vi "Tool Data.TestLauncher.vi"() -> ()   [LabVIEW 2019, in "Tool Data.lvclass"]
uses:
  Tool Data.lvclass
  <vilib>/JKI/JKI SMO/SMO/Typedefs/SMOState --Enum.ctl
  C:/Program Files (x86)/National Instruments/LabVIEW 2019/vi.lib/JKI/JKI SMO/SMO/SMO.lvclass
  Typedefs/PrivateEvents--Tool Data.Update Objects.ctl
  Settings/Setting Database/Typedefs/PublicEvents--Setting Database.PathsUpdated.ctl
  Settings/Path Settings/Path Settings.lvclass
  Settings/Setting Database/Typedefs/PublicEvents--Setting Database.RectanglesUpdated.ctl
  Settings/Rectangle Settings/Rectangle Settings.lvclass
  Settings/Setting Database/Typedefs/PublicEvents--Setting Database.FunnelsUpdated.ctl
  Settings/Funnel Settings/Funnel Settings.lvclass
  Settings/Setting Database/Typedefs/PublicEvents--Setting Database.DotsUpdated.ctl
  Settings/Dot Settings/Dot Settings.lvclass
  Parse/ParsePaths/Path.lvclass
  Parse/Rectangle/Rectangle.lvclass
  Parse/Image/SVGImage.lvclass
  Parse/Dot/Dot.lvclass
  <vilib>/JKI/JKI SMO/SMO/SMO.lvclass/SMO.ctl
  Tool Data.lvclass/Tool Data.ctl
  <vilib>/JKI/JKI SMO/SMO/Private/ReftoDVR--SMO.vi
  <vilib>/JKI/JKI SMO/SMO/SMO.lvclass
  Settings/Setting Database/Setting Database.lvclass
  Parse/PathCommands.Moveto/PathCommands.MoveTo.lvclass
  Parse/PathCommands.LineTo/PathCommands.LineTo.lvclass
  Parse/PathCommands.CurveTo/PathCommands.CurveTo.lvclass
  Parse/PathCommands.ClosePath/PathCommands.ClosePath.lvclass
  Parse/CSSProperties/CSSProperties.lvclass
  Parse/Transform.Translate/Transform.Translate.lvclass
  Parse/Transform.Matrix/Transform.Matrix.lvclass
panel:
  out "XY Graph":cluster{"X":dbl, "Y":dbl}[](graph)
  out "Paths":i32
  out "Rects":i32
  out "Funnels":i32
  out "Dots":i32
  in  "Send":bool
  out "SMO State":T1
  out "error out":errorcluster
  in  "Stop":bool
  # "Basic SMO Test Launcher"
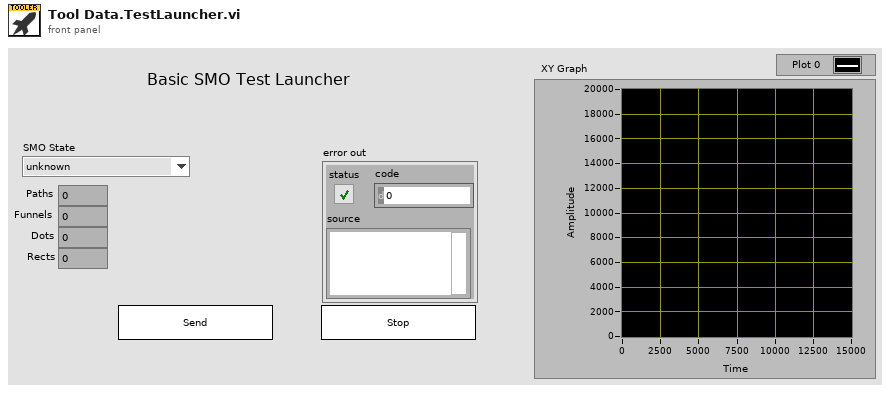
[diagram p1: front panel]
types:
  T1 = typedef "SMO.lvclass/SMOState --Enum.ctl" = enum16{"unknown", "Created", "Started", "Stopped"}
  T2 = typedef "Tool Data.lvclass/PrivateEvents--Tool Data.Update Objects.ctl" = cluster{"Settings":cluster{"Paths":T3, "Rectangles":T4, "Funnels":T5, "Dots":T6}, "Data":cluster{"Paths":refnum<class "Path.lvclass">[], "Rectangles":refnum<class "Rectangle.lvclass">[], "SVGImage":refnum<class "SVGImage.lvclass">, "Dots":refnum<class "Dot.lvclass">[], "Funnels":refnum<class "Path.lvclass">[]}}
  T3 = typedef "Setting Database.lvclass/PublicEvents--Setting Database.PathsUpdated.ctl" = refnum<class "Path Settings.lvclass">[]
  T4 = typedef "Setting Database.lvclass/PublicEvents--Setting Database.RectanglesUpdated.ctl" = refnum<class "Rectangle Settings.lvclass">[]
  T5 = typedef "Setting Database.lvclass/PublicEvents--Setting Database.FunnelsUpdated.ctl" = refnum<class "Funnel Settings.lvclass">[]
  T6 = typedef "Setting Database.lvclass/PublicEvents--Setting Database.DotsUpdated.ctl" = refnum<class "Dot Settings.lvclass">[]
  T7 = cluster{"Paths":T3, "Rectangles":T4, "Funnels":T5, "Dots":T6}
  T8 = cluster{"Paths":refnum<class "Path.lvclass">[], "Rectangles":refnum<class "Rectangle.lvclass">[], "SVGImage":refnum<class "SVGImage.lvclass">, "Dots":refnum<class "Dot.lvclass">[]}
  T9 = typedef "SMO.lvclass/Public Events.ctl" = cluster{"Error":refnum<user-event>, "State":refnum<user-event>, "Reserve State":refnum<user-event>}
  T10 = typedef "Tool Data.lvclass/PublicEvents--Cluster.ctl" = cluster{"Objects Updated":refnum<user-event>}
  T11 = cluster{"Event Registration Refnum":refnum<event-registration>}
  T12 = typedef "Relay-Box.lvclass/Resistor--enum.ctl" = enum16{"open", "discharge tip", "0 ohms", "100k ohm", "10M ohm", "1G ohm"}
  T13 = cluster{"Name":string, "Litho":cluster{"X":dbl, "Y":dbl, "Speed":dbl, "Voltage":dbl}[], "Set Resistance":T12, "Meta":variant}[]
  T14 = cluster{"X":dbl, "Y":dbl, "Speed":dbl, "Voltage":dbl}[]
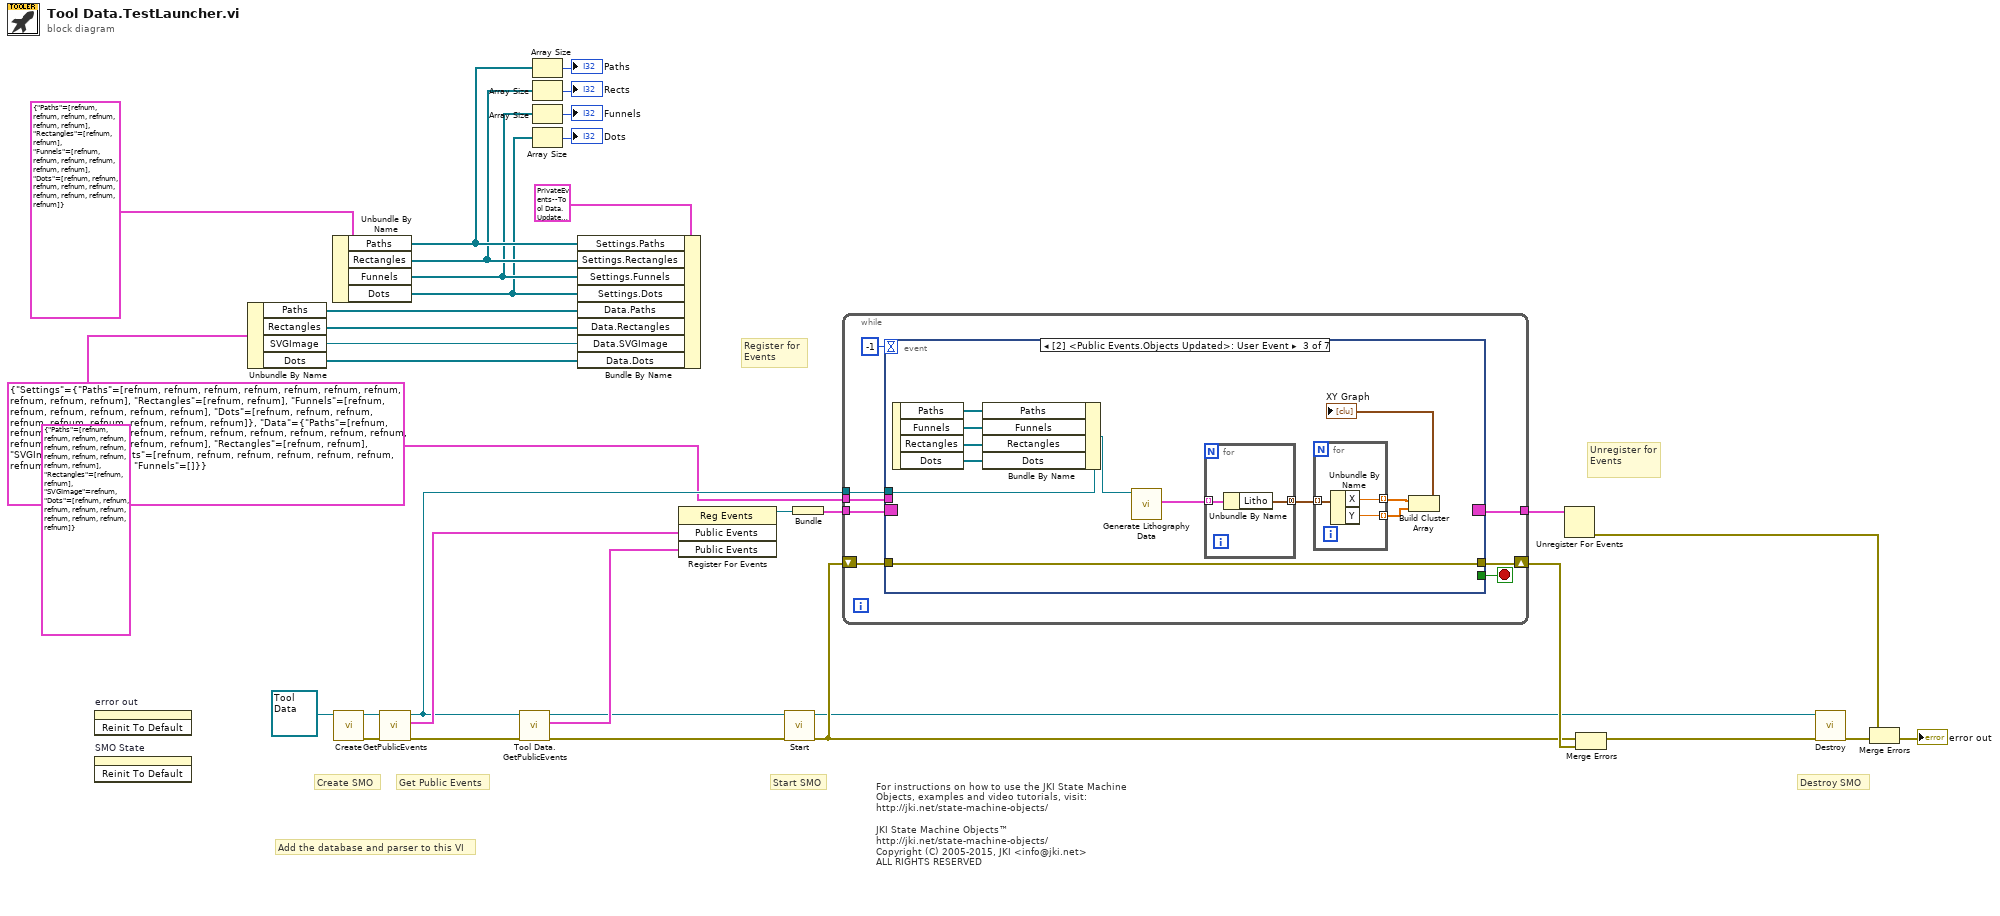
[diagram p0: block diagram]
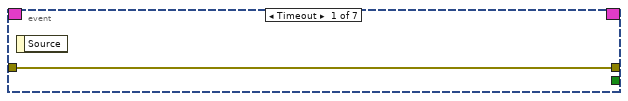
[diagram p2: hidden frame]
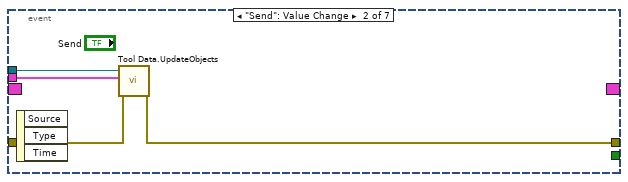
[diagram p3: hidden frame]
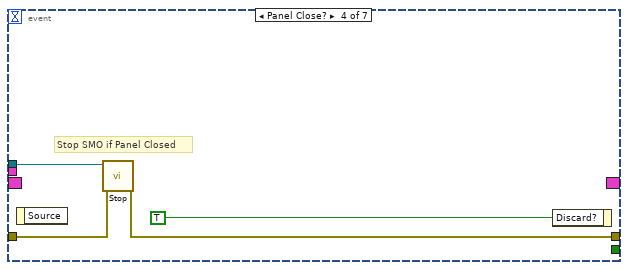
[diagram p4: hidden frame]
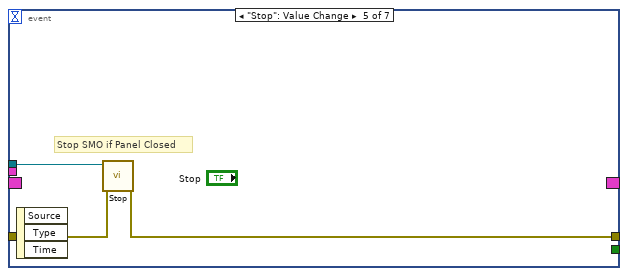
[diagram p5: hidden frame]
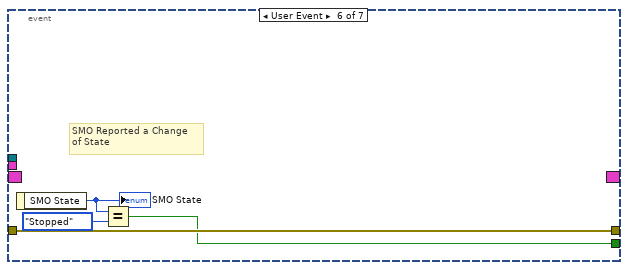
[diagram p6: hidden frame]
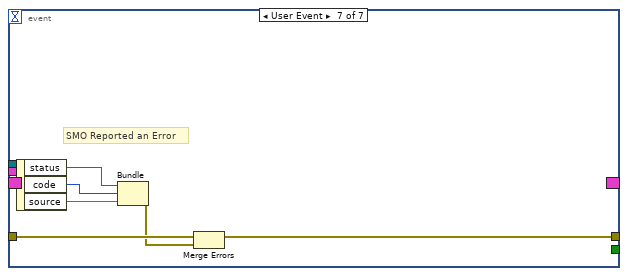
[diagram p7: hidden frame]
diagram:
  # "Add the database and parser to this VI"
  # "For instructions on how to use the JKI State Machine Objects, examples and video tutorials, visit:\nhttp://jki.net/state-machine-objects/\n\nJKI State Machine Objects™\nhttp://jki.net/state-machine-objects/\nCopyright (C) 2005-2015, JKI <info@jki.net>\nALL RIGHTS RESERVED"
  # "Get Public Events"
  # "Start SMO"
  # "Destroy SMO"
  # "Create SMO"
  # "Unregister for Events"
  # "Register for Events"
  n1 = invoke on="error out" class="Clust (strict)" method="Reinit To Default"() -> ()  [unwired: 3 in, 3 out]
  n2 = invoke on="SMO State" class="Enum (strict)" method="Reinit To Default"() -> ()  [unwired: 3 in, 3 out]
  n3 = Unbundle By Name(T8 {"Paths"=[refnum, refnum, refnum, refnum, refnum, refnum, refnum, refnum, refnum, refnum, refnum, refnum], "Rectangles"=[refnum, refnum], "SVGImage"=refnum, "Dots"=[refnum, refnum, refnum, refnum, refnum, refnum, refnum, refnum, refnum]}) -> ("Paths"=w13:refnum<class "Path.lvclass">[], "Rectangles"=w12:refnum<class "Rectangle.lvclass">[], "SVGImage"=w11:refnum<class "SVGImage.lvclass">, "Dots"=w10:refnum<class "Dot.lvclass">[])
  n4 = Unbundle By Name(T7 {"Paths"=[refnum, refnum, refnum, refnum, refnum, refnum], "Rectangles"=[refnum, refnum], "Funnels"=[refnum, refnum, refnum, refnum, refnum, refnum], "Dots"=[refnum, refnum, refnum, refnum, refnum, refnum, refnum, refnum, refnum]} ("Response")) -> ("Paths"=w9:T3, "Rectangles"=w8:T4, "Funnels"=w7:T5, "Dots"=w6:T6)
  n5 = call <vilib>:"Create.vi"("SMO"=refnum<class "Tool Data.lvclass"> refnum ("SMO.Template.lvclass")) -> ("error out"=w24:errorcluster, "SMO out"=w25:refnum<class "Tool Data.lvclass">)  [unwired: 8 in, 1 out]
  n6 = call <vilib>:"GetPublicEvents.vi"("error in (no error)"=w24, "SMO"=w25) -> ("error out"=w21:errorcluster, "Public Events"=w23:T9, "SMO out"=w18:refnum<class "Tool Data.lvclass">)  [unwired: 7 in]
  n7 = call "Tool Data.GetPublicEvents.vi"("error in (no error)"=w21, "Tool Data"=w18) -> ("error out"=w20:errorcluster, "Public Events"=w19:T10, "Tool Data out"=w17:refnum<class "Tool Data.lvclass">)  [unwired: 7 in]
  n8 = Array Size(array=w9) -> (size(s)=→"Paths":i32)
  n9 = Array Size(array=w8) -> (size(s)=→"Rects":i32)
  n10 = Array Size(array=w7) -> (size(s)=→"Funnels":i32)
  n11 = Array Size(array=w6) -> (size(s)=→"Dots":i32)
  n12 = Bundle By Name(cluster=T2 {"Settings"={"Paths"=[], "Rectangles"=[], "Funnels"=[], "Dots"=[]}, "Data"={"Paths"=[], "Rectangles"=[], "SVGImage"=refnum, "Dots"=[], "Funnels"=[]}} ("Updated Objects"), "Settings.Paths"=w9, "Settings.Rectangles"=w8, "Settings.Funnels"=w7, "Settings.Dots"=w6, "Data.Paths"=w13, "Data.Rectangles"=w12, "Data.SVGImage"=w11, "Data.Dots"=w10) -> ()  [unwired: 1 out]
  n13 = register-events(w23, w19) -> (reference out=w22:refnum<event-registration>)  [unwired: 2 in, 1 out]
  n14 = call <vilib>:"Start.vi"("error in (no error)"=w20, "SMO"=w17) -> ("error out"=w28:errorcluster, "SMO out"=w26:refnum<class "Tool Data.lvclass">)  [unwired: 8 in]
  n15 = Bundle("Event Registration Refnum"=w22) -> (w34:T11)  [unwired: 1 in]
  n16 = while {
    shift-right: [w42] -> w33
    shift-left: w28 -> [w41]
    tunnel: w34 -> [w40]
    tunnel: [w39] -> w35
    tunnel: w18 -> [w38]
    tunnel: T2 {"Settings"={"Paths"=[refnum, refnum, refnum, refnum, refnum, refnum, refnum, refnum, refnum, refnum], "Rectangles"=[refnum, refnum], "Funnels"=[refnum, refnum, refnum, refnum, refnum, refnum], "Dots"=[refnum, refnum, refnum, refnum, refnum, refnum, refnum, refnum, refnum]}, "Data"={"Paths"=[refnum, refnum, refnum, refnum, refnum, refnum, refnum, refnum, refnum, refnum, refnum, refnum, refnum, refnum, refnum, refnum], "Rectangles"=[refnum, refnum], "SVGImage"=refnum, "Dots"=[refnum, refnum, refnum, refnum, refnum, refnum, refnum, refnum, refnum], "Funnels"=[]}} ("Update Objects") -> [w36]
    stop <- w43 stop-if-true
    n17 = event shown="[2] <Public Events.Objects Updated>: User Event" {
      selector: w40 -> [_ _ _ _ _ _ _]
      dyn-events: [_ _ _ _ _ _ _] -> w39
      timeout: -1 -> [_ _ _ _ _ _ _]
      tunnel: [_ _ _ _ _ w73 _] -> w43
      tunnel: w38 -> [_ w48 w58 w69 w72 _ _]
      tunnel: [w44 w47 w60 w68 w71 w76 w80] -> w42
      tunnel: w41 -> [w44 w46 w60 w67 w70 w76 w78]
      tunnel: w36 -> [_ w45 _ _ _ _ _]
      event Timeout {
        n18 = event-data() -> ()  [unwired: 1 in, 1 out]
      }
      event "Send": Value Change {
        n19 = event-data() -> ()  [unwired: 1 in, 3 out]
        n20 = call "Tool Data.UpdateObjects.vi"("error in (no error)"=w46, "Updated Objects"=w45, "Tool Data"=w48) -> ("error out"=w47:errorcluster)  [unwired: 7 in, 1 out]
      }
      event User Event {
        n21 = event-data() -> ("Paths"=w57:refnum<class "Tool Path.lvclass">[], "Funnels"=w56:refnum<class "Tool Funnel.lvclass">[], "Rectangles"=w55:refnum<class "Tool Rectangle.lvclass">[], "Dots"=w54:refnum<class "Tool Dots.lvclass">[])  [unwired: 1 in]
        n22 = Bundle By Name(cluster=w58, "Paths"=w57, "Funnels"=w56, "Rectangles"=w55, "Dots"=w54) -> (w59:refnum<class "Tool Data.lvclass">)
        n23 = call-dynamic "Generate Lithography Data.vi"("Tool Data in"=w59) -> ("Lithography Data"=w53:T13)  [unwired: 8 in, 2 out]
        n24 = for {
          tunnel: w53 -> [w65] mode=indexing
          tunnel: [w64] -> w52 mode=concatenating
          n25 = Unbundle By Name(w65) -> ("Litho"=w64:T14)
        }
        n26 = for {
          tunnel: w52 -> [w63] mode=indexing
          tunnel: [w62] -> w51 mode=indexing
          tunnel: [w61] -> w50 mode=indexing
          n27 = Unbundle By Name(w63) -> ("X"=w62:dbl, "Y"=w61:dbl)
        }
        n28 = Build Cluster Array(w51, w50) -> (→"XY Graph":cluster{"X":dbl, "Y":dbl}[])
      }
      event Panel Close? {
        # "Stop SMO if Panel Closed"
        n29 = event-data() -> ()  [unwired: 1 in, 1 out]
        n30 = call <vilib>:"Stop.vi"("error in (no error)"=w67, "SMO"=w69) -> ("error out"=w68:errorcluster)  [unwired: 8 in, 1 out]
        n31 = event-data("Discard?"=TRUE ("OK")) -> ()  [unwired: 1 in, 1 out]
      }
      event "Stop": Value Change {
        # "Stop SMO if Panel Closed"
        n32 = event-data() -> ()  [unwired: 1 in, 3 out]
        n33 = call <vilib>:"Stop.vi"("error in (no error)"=w70, "SMO"=w72) -> ("error out"=w71:errorcluster)  [unwired: 8 in, 1 out]
      }
      event User Event {
        # "SMO Reported a Change\nof State"
        n34 = event-data() -> ("SMO State"=w75:T1)  [unwired: 1 in]
        "SMO State" <- w75
        n35 = Equal?(x=w75, y=SMOState_--Enum."Stopped") -> (x = y?=w73:bool)
      }
      event User Event {
        # "SMO Reported an Error"
        n36 = event-data() -> ("status"=w79:bool, "code"=w82:i32, "source"=w81:string)  [unwired: 1 in]
        n37 = Bundle("status"=w79, "code"=w82, "source"=w81) -> (w77:errorcluster)  [unwired: 1 in]
        n38 = Merge Errors(w78, w77) -> (w80:errorcluster)
      }
    }
  }
  n39 = Unregister For Events(event registration refnum=w35) -> (error out=w32:errorcluster)  [unwired: 1 in]
  n40 = Merge Errors(w28, w33) -> (w27:errorcluster)
  n41 = call <vilib>:"Destroy.vi"("error in (no error)"=w27, "SMO"=w26) -> ("error out"=w30:errorcluster)  [unwired: 9 in]
  n42 = Merge Errors(w32, w30) -> (→"error out":errorcluster)
